vi "High Resolution Relative Seconds.vi"(8 "error in (no error)":errorcluster) -> (0 "error out":errorcluster, 3 "relative seconds":dbl format="%_19f")   [LabVIEW 2016, in "SLL Debug.lvlib"]
doc: "High Resolution Relative Seconds with error in and error out"
uses:
  SLL Debug.lvlib
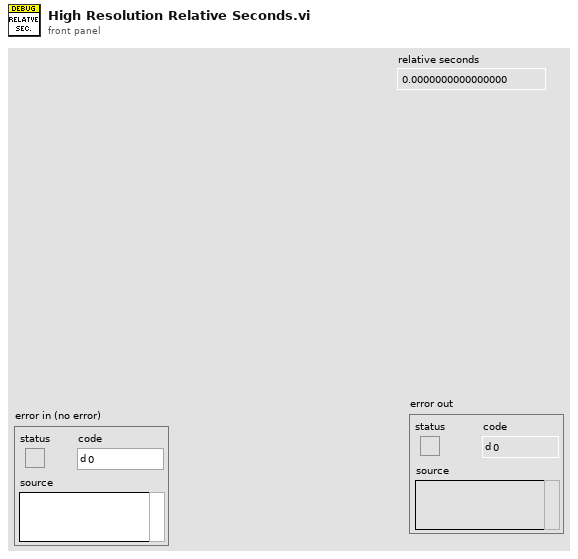
[diagram p1: front panel]
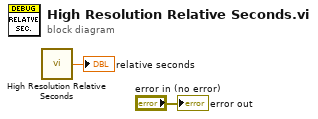
[diagram p0: block diagram]
diagram:
  n1 = call <vilib>:"High Resolution Relative Seconds.vi"() -> ("relative seconds"=→"relative seconds":dbl)
  "error out" <- "error in (no error)"
